vi "compute eqn and plot graph.vi"() -> ()   [LabVIEW 2024]
panel:
  out "y1":dbl[](array[numeric])
  out "y2":dbl[](array[numeric])
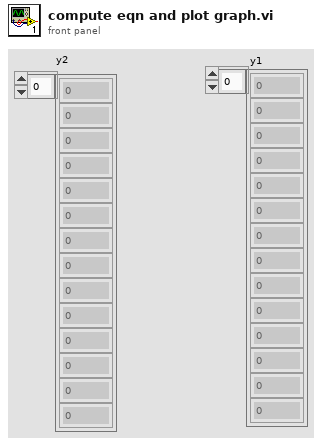
[diagram p1: front panel]
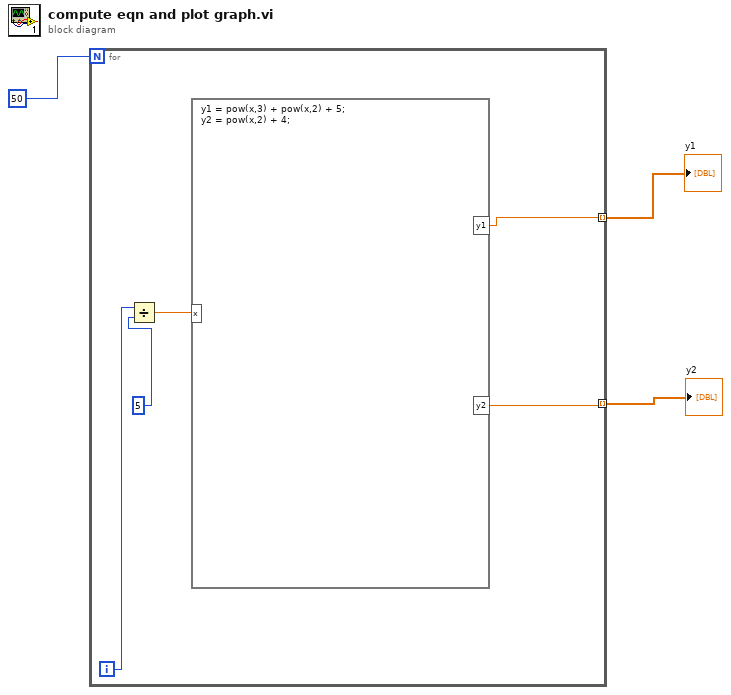
[diagram p0: block diagram]
diagram:
  n1 = for {
    N: 50 -> [_]
    tunnel: [w5] -> w2 mode=indexing
    tunnel: [w4] -> w1 mode=indexing
    i -> [w7]
    n2 = Divide(x=w7, y=5) -> (x/y=w8:dbl)
    n3 = formula code="y1 = pow(x,3) + pow(x,2) + 5;\ny2 = pow(x,2) + 4;"("x"=w8) -> ("y1"=w4:dbl, "y2"=w5:dbl)
  }
  "y2" <- w2
  "y1" <- w1
